vi "Set Kinetic Cycle Time.vi"(8 "error in (no error)":errorcluster, 11 "time":sgl) -> (0 "error out":errorcluster, 3 "function return":u32)   [LabVIEW 2018, in "AndorSDK.lvlib"]
doc: "EXPNETTYPE unsigned int WINAPI SetKineticCycleTime(float time);"
uses:
  AndorSDK.lvlib
  ATMCD32D.dll
  OwnVIs/AndorOWN.lvlib
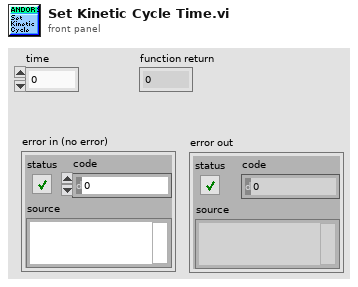
[diagram p1: front panel]
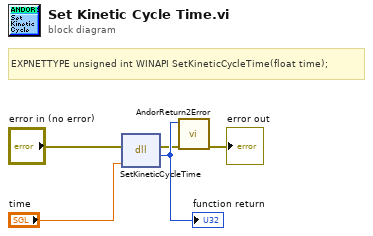
[diagram p0: block diagram]
diagram:
  # "EXPNETTYPE unsigned int WINAPI SetKineticCycleTime(float time);"
  n1 = dll-call lib="C:/Users/johan/Downloads/LabVIEW software/LabVIEW software/IX-81 Software/lib/ANDOR/Andor SDK/ATMCD32D.*" fn="SetKineticCycleTime"(error in="error in (no error)", "time"="time") -> (error out=w2:errorcluster, w3:u32)  [unwired: 3 in, 1 out]
  "function return" <- w3
  n2 = call "AndorReturn2Error.vi"("error in (no error)"=w2, "Camera return"=w3) -> ("error out"=→"error out":errorcluster)  [unwired: 9 in]
